vi "GlobalIFlatImgHndl.vi"() -> ()   [LabVIEW 2010]
panel:
  in  "Flat Active data":bool
  in  "Flat Image Handle":u32
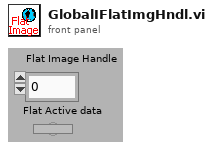
[diagram p1: front panel]
diagram:
